vi "LvDataToString.vi"(8 "error in (no error)":errorcluster, 11 "Variant":variant) -> (0 "error out":errorcluster, 3 "String Value":string)   [LabVIEW 2014, in "TableLogger_Actor.lvlib" / "TableLogger_Actor.lvclass"]
uses:
  TableLogger_Actor.lvclass
panel:
  # "Connector Pane"
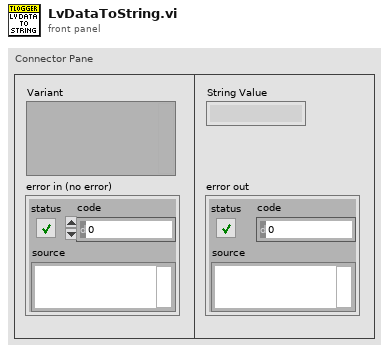
[diagram p1: front panel]
types:
  T1 = typedef "Type Descriptor Enumeration__ogtk.ctl" = enum8{"<Null>", "I8", "I16", "I32", "I64", "U8", "U16", "U32", "U64", "SGL", "DBL", "EXT", "CSG", "CDB", "CXT", "0x0F", "0x10", "0x11", "0x12", "0x13", "0x14", "Enum U8", "Enum U16", "Enum U32", "Enum U64", "SGL PQ", "DBL PQ", "EXT PQ", "CSG PQ", "CDB PQ", "CXT PQ", "0x1F", "0x20", "Boolean", "0x22", "0x23", "0x24", "0x25", "0x26", "0x27", "0x28", "0x29", "0x2A", "0x2B", "0x2C", "0x2D", "0x2E", "0x2F", "String", "0x31", "Path", "Pict", "0x34", "0x35", "0x36", "DAQ", "0x38", "0x39", "0x3A", "0x3B", "0x3C", "0x3D", "0x3E", "0x3F", "Array", "0x41", "0x42", "0x43", "0x44", "0x45", "0x46", "0x47", "0x48", "0x49", "0x4A", "0x4B", "0x4C", "0x4D", "0x4E", "0x4F", "Cluster", "0x51", "0x52", "Variant", "Waveform", "0x55", "0x56", "0x57", "0x58", "0x59", "0x5A", "0x5B", "0x5C", "0x5D", "0x5E", "0x5F", "0x60", "0x61", "0x62", "0x63", "0x64", "0x65", "0x66", "0x67", "0x68", "0x69", "0x6A", "0x6B", "0x6C", "0x6D", "0x6E", "0x6F", "Refnum"}
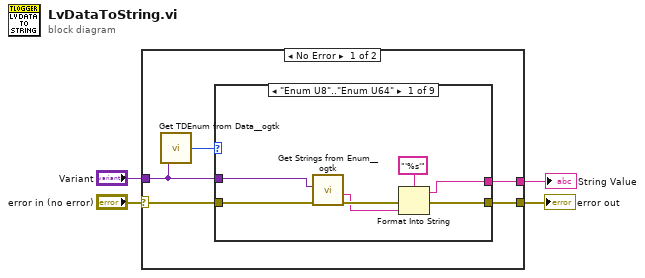
[diagram p0: block diagram]
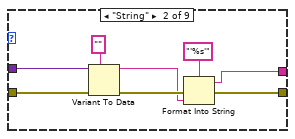
[diagram p2: hidden frame]
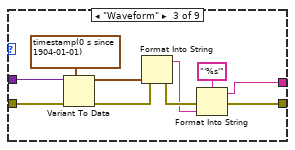
[diagram p3: hidden frame]
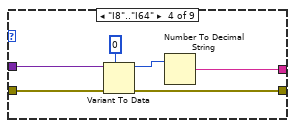
[diagram p4: hidden frame]
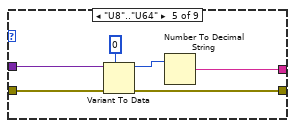
[diagram p5: hidden frame]
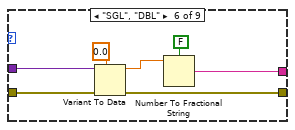
[diagram p6: hidden frame]
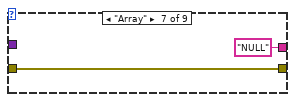
[diagram p7: hidden frame]
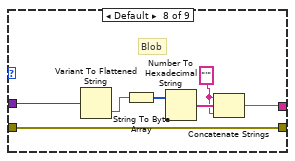
[diagram p8: hidden frame]
diagram:
  n1 = case shown="No Error" "error in (no error)" {
    selector: "error in (no error)" -> [w8 w64]
    tunnel: [w9 w64] -> w4
    tunnel: [w7 _] -> w2
    tunnel: "Variant" -> [w6 _]
    frame No Error {
      n2 = call <userlib>:"Get TDEnum from Data__ogtk.vi"("Data"=w6) -> ("Type Descriptor Enumeration"=w5:T1)  [unwired: 4 in]
      n3 = case shown="\"Enum U8\"..\"Enum U64\"" w5 {
        tunnel: [w12 w19 w27 w36 w42 w49 "NULL" ("String Value") w58 _] -> w7
        tunnel: w8 -> [w16 w24 w34 w40 w46 w53 w55 w57 w63]
        tunnel: w6 -> [w15 w23 w33 w39 w45 w52 _ w62 _]
        tunnel: [w13 w20 w28 w35 w41 w47 w55 w57 w63] -> w9
        frame "Enum U8".."Enum U64" {
          n4 = call <userlib>:"Get Strings from Enum__ogtk.vi"("error in (no error)"=w16, "Enum"=w15) -> ("error out"=w14:errorcluster, "String Value"=w11:string)  [unwired: 6 in, 2 out]
          n5 = Format Into String(format string="'%s'", error in=w14, w11) -> (resulting string=w12:string, error out=w13:errorcluster)  [unwired: 1 in]
        }
        frame "String" {
          n6 = Variant To Data(error in=w24, type="", Variant=w23) -> (data=w18:string, error out=w21:errorcluster)
          n7 = Format Into String(format string="'%s'", error in=w21, w18) -> (resulting string=w19:string, error out=w20:errorcluster)  [unwired: 1 in]
        }
        frame "Waveform" {
          n8 = Variant To Data(error in=w34, type=timestamp(0 s since 1904-01-01), Variant=w33) -> (data=w31:timestamp, error out=w30:errorcluster)
          n9 = Format Into String(error in=w30, w31) -> (resulting string=w26:string, error out=w29:errorcluster)  [unwired: 2 in]
          n10 = Format Into String(format string="'%s'", error in=w29, w26) -> (resulting string=w27:string, error out=w28:errorcluster)  [unwired: 1 in]
        }
        frame "I8".."I64" {
          n11 = Variant To Data(error in=w40, type=i64 0, Variant=w39) -> (data=w37:i64, error out=w35:errorcluster)
          n12 = Number To Decimal String(number=w37) -> (decimal integer string=w36:string)  [unwired: 1 in]
        }
        frame "U8".."U64" {
          n13 = Variant To Data(error in=w46, type=u64 0, Variant=w45) -> (data=w43:u64, error out=w41:errorcluster)
          n14 = Number To Decimal String(number=w43) -> (decimal integer string=w42:string)  [unwired: 1 in]
        }
        frame "SGL", "DBL" {
          n15 = Variant To Data(error in=w53, type=0.0, Variant=w52) -> (data=w50:dbl, error out=w47:errorcluster)
          n16 = Number To Fractional String(use system decimal point (T)=FALSE, number=w50) -> (F-format string=w49:string)  [unwired: 2 in]
        }
        frame "Array" {
        }
        frame Default {
          w56 = "'"
          # "Blob"
          n17 = Variant To Flattened String(Variant=w62) -> (data string=w61:string)  [unwired: 1 out]
          n18 = String To Byte Array(string=w61) -> (unsigned byte array=w60:u8[])
          n19 = Number To Hexadecimal String(2:w60) -> (0:w59:string[])  [unwired: 1 in]
          n20 = Concatenate Strings(w56, w59, w56) -> (w58:string)
        }
        frame "Cluster" {
        }
      }
    }
    frame Error {
    }
  }
  "error out" <- w4
  "String Value" <- w2
